vi "Get Quantity.vi"(6 "Backend engine":T2, 8 "error in":errorcluster, 11 "Quantity Name":string) -> (0 "error out":errorcluster, 3 "Quantity":T1)   [LabVIEW 2013, in "QWTBLVLib.lvlib"]
doc: "Get Quantity."
uses:
  QWTBLVLib.lvlib
  TD Backend Engine.ctl
  TD Quantity.ctl
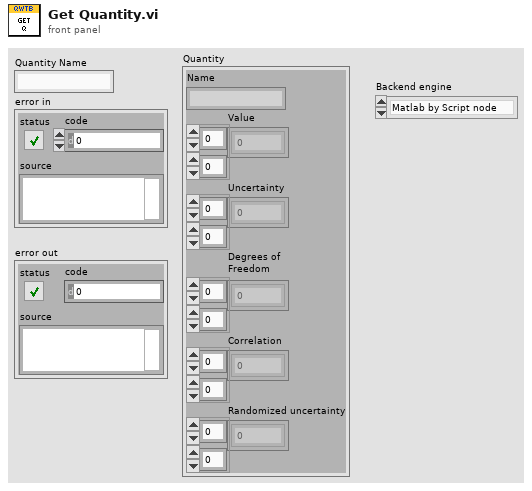
[diagram p1: front panel]
types:
  T1 = typedef "QWTBLVLib.lvlib/TD Quantity.ctl" = cluster{"Name":string, "Value":dbl[][], "Uncertainty":dbl[][], "Degrees of\nFreedom":dbl[][], "Correlation":dbl[][], "Randomized uncertainty":dbl[][]}
  T2 = typedef "QWTBLVLib.lvlib/TD Backend Engine.ctl" = enum16{"Matlab by Script node", "GNU Octave by GOLPI"}
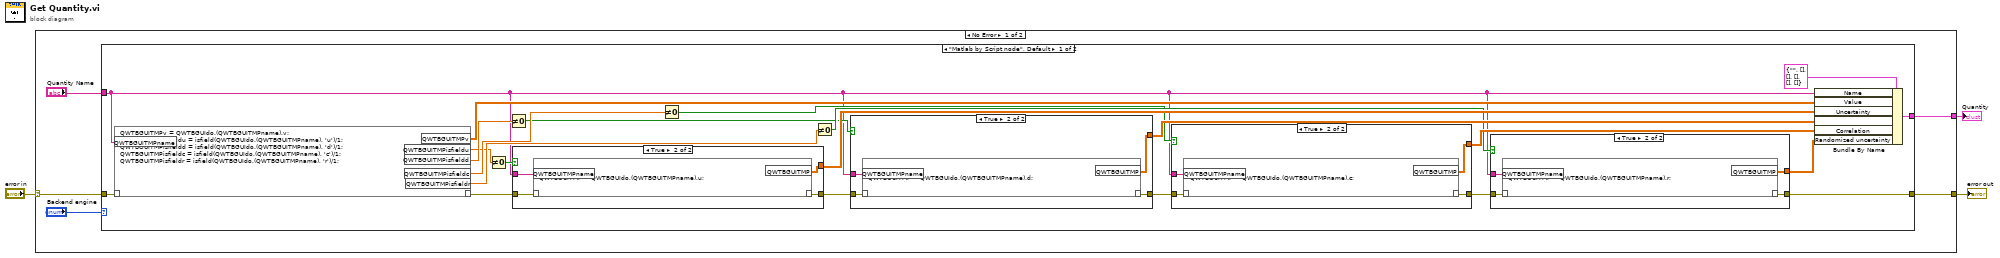
[diagram p0: block diagram]
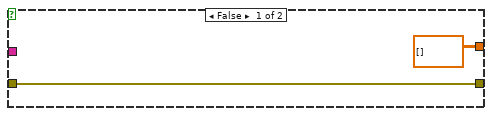
[diagram p2: hidden frame]
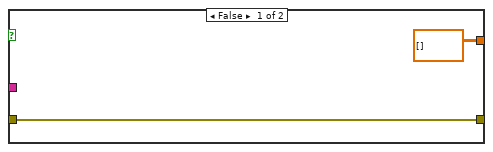
[diagram p3: hidden frame]
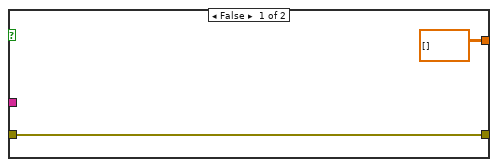
[diagram p4: hidden frame]
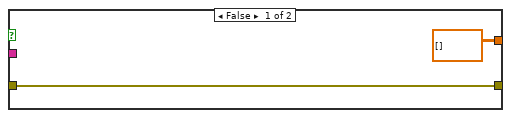
[diagram p5: hidden frame]
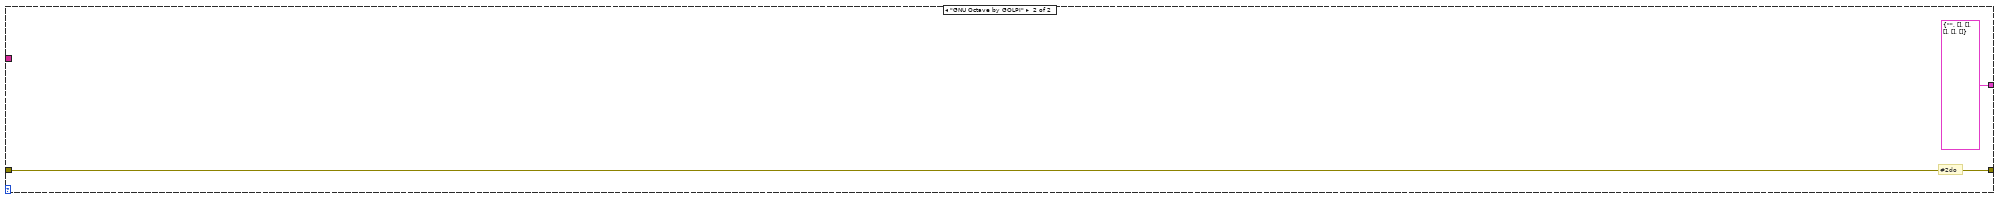
[diagram p6: hidden frame]
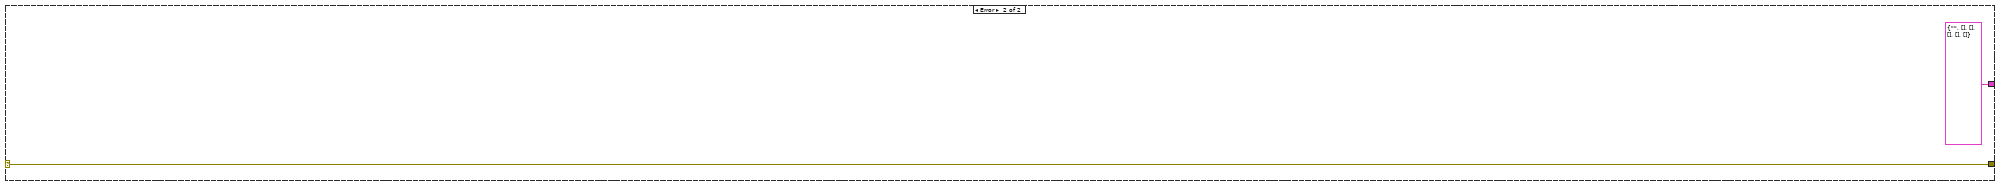
[diagram p7: hidden frame]
diagram:
  n1 = case shown="No Error" "error in" {
    selector: "error in" -> [w6 w58]
    tunnel: [w5 w58] -> w3
    tunnel: [w7 T1 {"Name"="", "Value"=[], "Uncertainty"=[], "Degrees of\nFreedom"=[], "Correlation"=[], "Randomized uncertainty"=[]} ("Quantity")] -> w1
    frame No Error {
      n2 = case shown="\"Matlab by Script node\", Default" "Backend engine" {
        tunnel: "Quantity Name" -> [w13 _]
        tunnel: [w11 T1 {"Name"="", "Value"=[], "Uncertainty"=[], "Degrees of\nFreedom"=[], "Correlation"=[], "Randomized uncertainty"=[]} ("Quantity")] -> w7
        tunnel: w6 -> [w10 w55]
        tunnel: [w9 w55] -> w5
        frame "Matlab by Script node", Default {
          n3 = script code="QWTBGUITMPv = QWTBGUIdo.(QWTBGUITMPname).v;\nQWTBGUITMPisfieldu = isfield(QWTBGUIdo.(QWTBGUITMPname), 'u')/1;\nQWTBGUITMPisfieldd = isfield(QWTBGUIdo.(QWTBGUITMPname), 'd')/1;\nQWTBGUITMPisfieldc = isfield(QWTBGUIdo.(QWTBGUITMPname), 'c')/1;\nQWTBGUITMPisfieldr = isfield(QWTBGUIdo.(QWTBGUITMPname), 'r')/1;"("??"=w10, "QWTBGUITMPname"=w13) -> ("??"=w16:errorcluster, "QWTBGUITMPv"=w26:dbl[][], "QWTBGUITMPisfieldu"=w14:dbl, "QWTBGUITMPisfieldd"=w18:dbl, "QWTBGUITMPisfieldc"=w22:dbl, "QWTBGUITMPisfieldr"=w24:dbl)
          n4 = Not Equal To 0?(x=w14) -> (x != 0?=w15:bool)
          n5 = Not Equal To 0?(x=w18) -> (x != 0?=w19:bool)
          n6 = case shown="True" w15 {
            tunnel: w16 -> [w50 w54]
            tunnel: [w50 w53] -> w17
            tunnel: [dbl[][] [] w52] -> w27
            tunnel: w13 -> [_ w51]
            frame False {
            }
            frame True {
              n7 = script code="QWTBGUITMP = QWTBGUIdo.(QWTBGUITMPname).u;"("??"=w54, "QWTBGUITMPname"=w51) -> ("??"=w53:errorcluster, "QWTBGUITMP"=w52:dbl[][])
            }
          }
          n8 = Not Equal To 0?(x=w22) -> (x != 0?=w23:bool)
          n9 = Not Equal To 0?(x=w24) -> (x != 0?=w25:bool)
          n10 = case shown="True" w19 {
            tunnel: w17 -> [w44 w48]
            tunnel: [w44 w47] -> w20
            tunnel: [dbl[][] [] w46] -> w28
            tunnel: w13 -> [_ w45]
            frame False {
            }
            frame True {
              n11 = script code="QWTBGUITMP = QWTBGUIdo.(QWTBGUITMPname).d;"("??"=w48, "QWTBGUITMPname"=w45) -> ("??"=w47:errorcluster, "QWTBGUITMP"=w46:dbl[][])
            }
          }
          n12 = case shown="True" w23 {
            tunnel: w20 -> [w38 w42]
            tunnel: [w38 w41] -> w21
            tunnel: [dbl[][] [] w40] -> w29
            tunnel: w13 -> [_ w39]
            frame False {
            }
            frame True {
              n13 = script code="QWTBGUITMP = QWTBGUIdo.(QWTBGUITMPname).c;"("??"=w42, "QWTBGUITMPname"=w39) -> ("??"=w41:errorcluster, "QWTBGUITMP"=w40:dbl[][])
            }
          }
          n14 = case shown="True" w25 {
            tunnel: w21 -> [w32 w36]
            tunnel: [w32 w35] -> w9
            tunnel: [dbl[][] [] w34] -> w30
            tunnel: w13 -> [_ w33]
            frame False {
            }
            frame True {
              n15 = script code="QWTBGUITMP = QWTBGUIdo.(QWTBGUITMPname).r;"("??"=w36, "QWTBGUITMPname"=w33) -> ("??"=w35:errorcluster, "QWTBGUITMP"=w34:dbl[][])
            }
          }
          n16 = Bundle By Name(cluster=T1 {"Name"="", "Value"=[], "Uncertainty"=[], "Degrees of\nFreedom"=[], "Correlation"=[], "Randomized uncertainty"=[]} ("Quantity"), "Name"=w13, "Value"=w26, "Uncertainty"=w27, "Degrees of\nFreedom"=w28, "Correlation"=w29, "Randomized uncertainty"=w30) -> (w11:T1)
        }
        frame "GNU Octave by GOLPI" {
          # "#2do"
        }
      }
    }
    frame Error {
    }
  }
  "error out" <- w3
  "Quantity" <- w1
